vi "Function of Time Global.vi"() -> ()   [LabVIEW 2012]
panel:
  in  "Elapsed Time":dbl
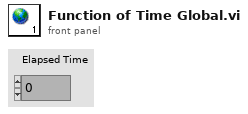
[diagram p1: front panel]
diagram:
